vi "Setup subWorker - TCP Server.vi"(8 "error in":errorcluster, 11 "TCP Server Example in":refnum<class "TCP Server Example.lvclass">) -> (0 "error out":errorcluster, 3 "TCP Server Example out":refnum<class "TCP Server Example.lvclass">)   [LabVIEW 2017, in "TCP Server Example.lvclass"]
doc: "This VI sets up the framework parameters of a statically-linked subWorker."
uses:
  TCP Server Example.lvclass
  TCP Server Example.lvclass/TCP Server Example.ctl
  TCP Server/TCP Server/TCP Server.lvclass
  C:/SC/Source Code/VIPM/LabVIEW 20xx/vi.lib/addons/_Workers/Library/Classes/Worker/Worker.lvclass
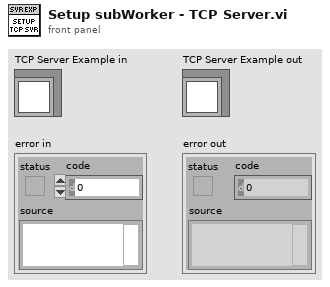
[diagram p1: front panel]
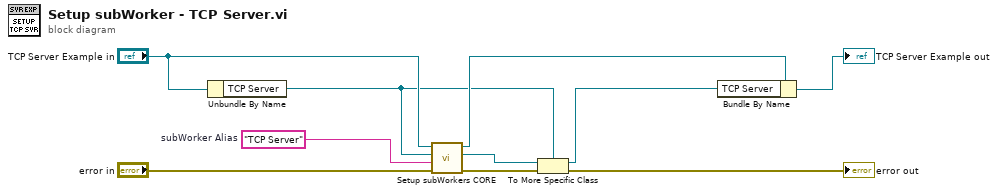
[diagram p0: block diagram]
diagram:
  w6 = "TCP Server"  # subWorker Alias
  n1 = Unbundle By Name("TCP Server Example in") -> ("TCP Server"=w3:refnum<class "TCP Server.lvclass">)
  n2 = call-dynamic "Setup subWorkers CORE.vi"("error in"="error in", "subWorker Alias"=w6, "subWorker"=w3, "Worker"="TCP Server Example in") -> ("error out"=w5:errorcluster, "subWorker out"=w1:refnum<class "Worker.lvclass">, "Worker out"=w8:refnum<class "TCP Server Example.lvclass">)  [unwired: 5 in]
  n3 = To More Specific Class(target class=w3, reference=w1, error in=w5) -> (specific class reference=w2:refnum<class "TCP Server.lvclass">, error out=→"error out":errorcluster)
  n4 = Bundle By Name(cluster=w8, "TCP Server"=w2) -> (→"TCP Server Example out":refnum<class "TCP Server Example.lvclass">)
